vi "GraphsSandbox.vi"() -> ()   [LabVIEW 2016]
uses:
  <vilib>/Utility/miscctls.llb/LVOffsetAndMultiplierTypeDef.ctl
  <vilib>/measure/maresamp.llb/Resample Pair of Arrays (single shot).vi
  <userlib>/_OpenG.lib/array/array.llb/Empty 1D Array (DBL)__ogtk.vi
  <vilib>/measure/NI_MAPro.lvlib
  <vilib>/Analysis/NI_AALPro.lvlib
panel:
  in  "dt":dbl=1.0 format="%.2p"
  out "XY graphs 2":cluster{dbl[], dbl[]}[](graph)
  out "Numeric":i32
  out "antisymmetric":cluster{dbl[], dbl[]}[](graph)
  out "symmetric":cluster{dbl[], dbl[]}[](graph)
  out "line cuts":cluster{dbl[], dbl[]}[](graph)
  in  "y values to make line cuts":dbl[](array[numeric]) format="%#_6p"
  out "resampled intensity graph":dbl[][](graph)
  in  "XY graphs":cluster{dbl[], dbl[]}[](graph)
  in  "\"y\" array (each curve's parameter)":dbl[](array[numeric])=[1.0] format="%#_6p"
  # "1. convert x and y arrays to x and y scales for intensity graph"
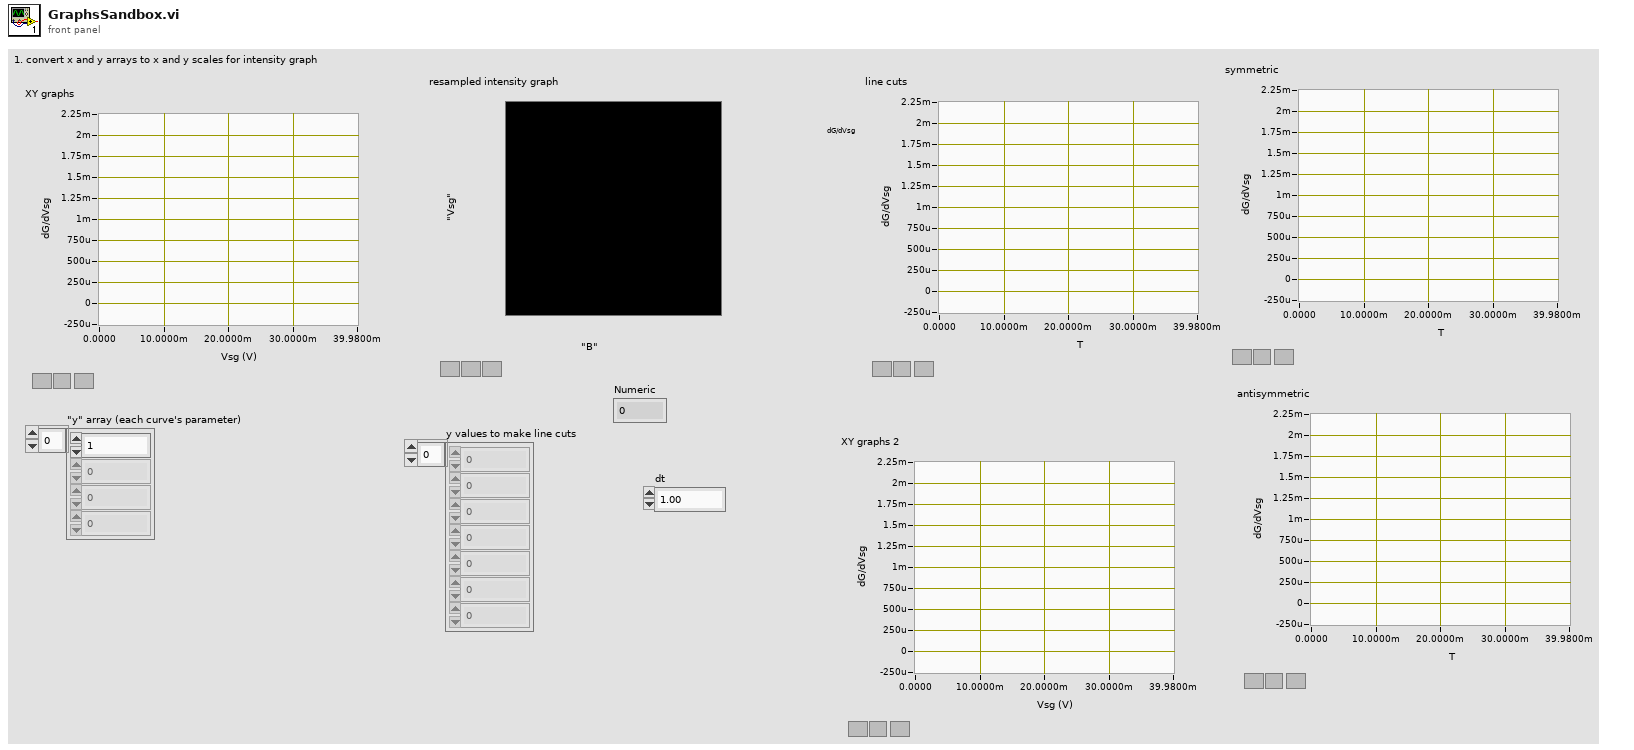
[diagram p1: front panel]
types:
  T1 = cluster{"x array":dbl[], "\"y\" array (parms)":dbl[], "XY graphs":cluster{dbl[], dbl[]}[]}
  T2 = typedef "LVOffsetAndMultiplierTypeDef.ctl" = cluster{"Offset":dbl, "Multiplier":dbl}
  T3 = cluster{"Decimated Array":dbl[], "Decimated Array":dbl[]}
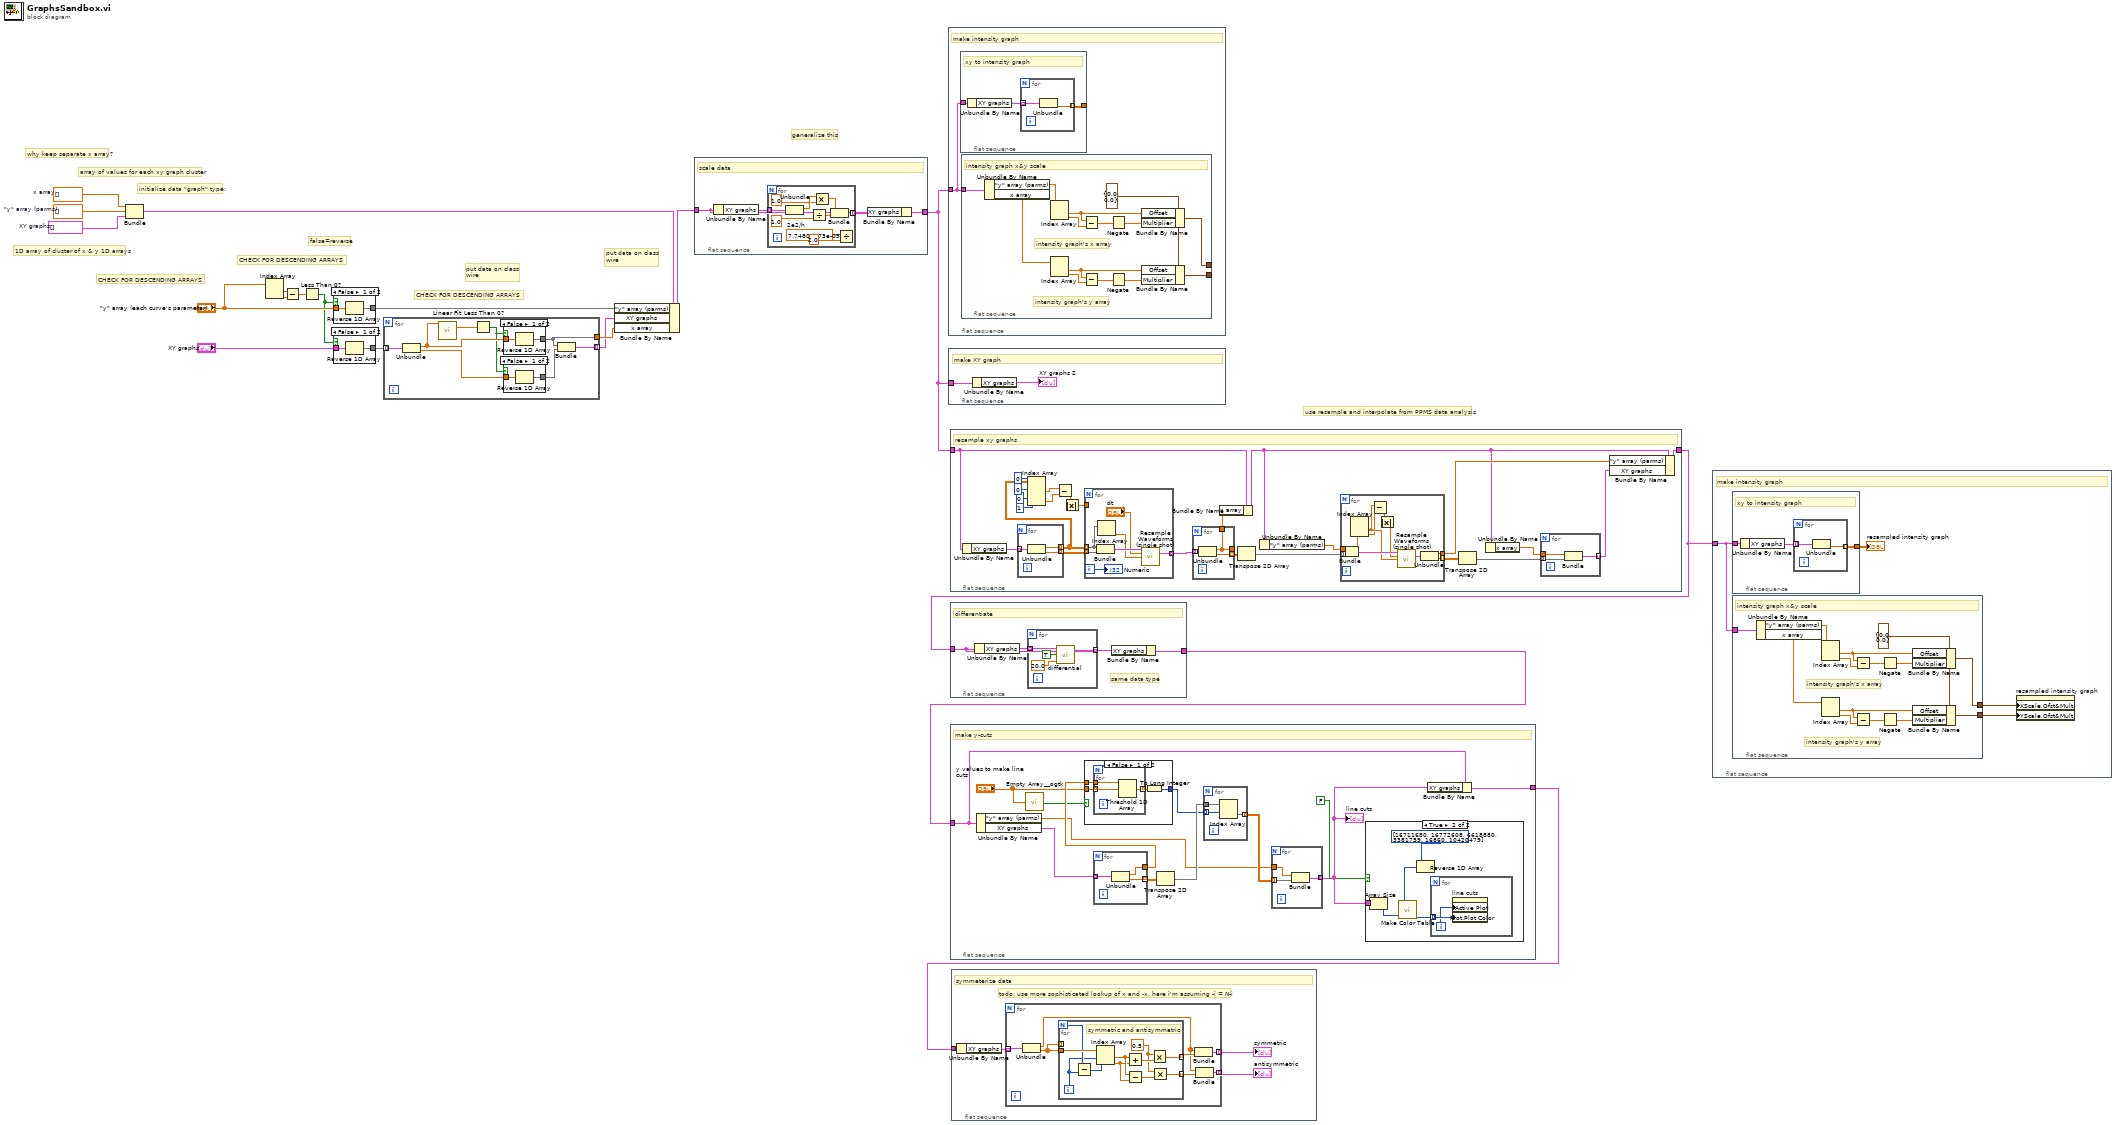
[diagram p0: block diagram]
diagram:
  w18 = dbl[] []  # x array
  w17 = cluster{dbl[], dbl[]}[] []  # XY graphs
  w19 = dbl[] []  # "y" array (parms)
  # "use resample and interpolate from PPMS data analysis"
  # "generalize this"
  # "array of values for each xy graph cluster"
  # "1D array of cluster of x & y 1D arrays"
  # "why keep separate x array?"
  # "CHECK FOR DESCENDING ARRAYS"
  # "false=reverse"
  # "put data on class\nwire"
  # "CHECK FOR DESCENDING ARRAYS"
  # "initialize data \"graph\" type:"
  # "CHECK FOR DESCENDING ARRAYS"
  # "put data on class\nwire"
  n1 = Bundle("x array"=w18, "\"y\" array (parms)"=w19, "XY graphs"=w17) -> (w16:T1)  [unwired: 1 in]
  n2 = Index Array(array="\"y\" array (each curve's parameter)") -> (element #1=w13:dbl, element #2=w14:dbl)  [unwired: 2 in]
  n3 = Subtract(x=w13, y=w14) -> (x-y=w12:dbl)
  n4 = Less Than 0?(x=w12) -> (x < 0?=w5:bool)
  n5 = case shown="False" w5 {
    tunnel: [w21 w22] -> w15
    tunnel: "\"y\" array (each curve's parameter)" -> [w20 w22]
    frame False {
      n6 = Reverse 1D Array(array=w20) -> (reversed array=w21:dbl[])
    }
    frame True {
    }
  }
  n7 = case shown="False" w5 {
    tunnel: [w24 w25] -> w6
    tunnel: "XY graphs" -> [w23 w25]
    frame False {
      n8 = Reverse 1D Array(array=w23) -> (reversed array=w24:cluster{dbl[], dbl[]}[])
    }
    frame True {
    }
  }
  n9 = for {
    tunnel: w6 -> [w33] mode=indexing
    tunnel: [w32] -> w10 mode=indexing
    tunnel: [w26] -> w11
    n10 = Unbundle(w33) -> (w30:dbl[], w28:dbl[])
    n11 = call <vilib>:"Linear Fit.vi"("Y"=w30) -> ("slope"=w31:dbl)  [unwired: 10 in, 4 out]
    n12 = Less Than 0?(x=w31) -> (x < 0?=w29:bool)
    n13 = case shown="False" w29 {
      tunnel: [w38 w39] -> w26
      tunnel: w30 -> [w37 w39]
      frame False {
        n14 = Reverse 1D Array(array=w37) -> (reversed array=w38:dbl[])
      }
      frame True {
      }
    }
    n15 = case shown="False" w29 {
      tunnel: [w35 w36] -> w27
      tunnel: w28 -> [w34 w36]
      frame False {
        n16 = Reverse 1D Array(array=w34) -> (reversed array=w35:dbl[])
      }
      frame True {
      }
    }
    n17 = Bundle(w26, w27) -> (w32:cluster{dbl[], dbl[]})  [unwired: 1 in]
  }
  n18 = Bundle By Name(cluster=w16, "\"y\" array (parms)"=w15, "XY graphs"=w10, "x array"=w11) -> (w9:T1)
  n19 = flat-sequence {
    tunnel: w9 -> [w41]
    tunnel: [w40] -> w4
    frame #0 {
      # "scale data"
      n20 = Unbundle By Name(w41) -> ("XY graphs"=w43:cluster{dbl[], dbl[]}[])
      n21 = for {
        tunnel: w43 -> [w53] mode=indexing
        tunnel: [w48] -> w42 mode=indexing
        w47 = 7.74809173e-05  # 2e2/h
        n22 = Unbundle(w53) -> (w50:dbl[], w52:dbl[])
        n23 = Divide(x=w52, y=1.0) -> (x/y=w51:dbl[])
        n24 = Multiply(x=w50, y=1.0) -> (x*y=w45:dbl[])
        n25 = Bundle(w45, w51) -> (w48:cluster{dbl[], dbl[]})  [unwired: 1 in]
        n26 = Divide(x=w47, y=2.0) -> ()  [unwired: 1 out]
      }
      n27 = Bundle By Name(cluster=w41, "XY graphs"=w42) -> (w40:T1)
    }
  }
  n28 = flat-sequence {
    tunnel: w4 -> [w54]
    frame #0 {
      # "make intensity graph"
      n29 = flat-sequence {
        tunnel: w54 -> [w70]
        tunnel: [w69] -> _
        frame #0 {
          # "xy to intensity graph"
          n30 = Unbundle By Name(w70) -> ("XY graphs"=w71:cluster{dbl[], dbl[]}[])
          n31 = for {
            tunnel: w71 -> [w73] mode=indexing
            tunnel: [w72] -> w69 mode=indexing
            n32 = Unbundle(w73) -> (w72:dbl[])  [unwired: 1 out]
          }
        }
      }
      n33 = flat-sequence {
        tunnel: [w68] -> _
        tunnel: [w58] -> _
        tunnel: w54 -> [w55]
        frame #0 {
          w59 = T2 {"Offset"=0.0, "Multiplier"=0.0} ("X Scale.Offset and Multiplier")
          # "intensity graph's y array"
          # "intensity graph's x array"
          # "intensity graph x&y scale"
          n34 = Unbundle By Name(w55) -> ("\"y\" array (parms)"=w57:dbl[], "x array"=w56:dbl[])
          n35 = Index Array(array=w57) -> (element #1=w62:dbl, element #2=w67:dbl)  [unwired: 2 in]
          n36 = Index Array(array=w56) -> (element #1=w60:dbl, element #2=w64:dbl)  [unwired: 2 in]
          n37 = Subtract(x=w62, y=w67) -> (x-y=w66:dbl)
          n38 = Subtract(x=w60, y=w64) -> (x-y=w65:dbl)
          n39 = Negate(x=w66) -> (-x=w63:dbl)
          n40 = Negate(x=w65) -> (-x=w61:dbl)
          n41 = Bundle By Name(cluster=w59, "Offset"=w62, "Multiplier"=w63) -> (w68:T2)
          n42 = Bundle By Name(cluster=w59, "Offset"=w60, "Multiplier"=w61) -> (w58:T2)
        }
      }
    }
  }
  n43 = flat-sequence {
    tunnel: w4 -> [w74]
    frame #0 {
      # "make XY graph"
      n44 = Unbundle By Name(w74) -> ("XY graphs"=→"XY graphs 2":cluster{dbl[], dbl[]}[])
    }
  }
  n45 = flat-sequence {
    tunnel: [w91] -> w2
    tunnel: w4 -> [w78]
    frame #0 {
      # "resample xy graphs"
      n46 = Unbundle By Name(w78) -> ("XY graphs"=w90:cluster{dbl[], dbl[]}[])
      n47 = for {
        tunnel: w90 -> [w102] mode=indexing
        tunnel: [w101] -> w89 mode=indexing
        tunnel: [w100] -> w84 mode=indexing
        n48 = Unbundle(w102) -> (w100:dbl[], w101:dbl[])
      }
      n49 = Index Array(array=w84, index (row) #1=0 ("index (row)"), index (col) #1=0 ("disabled index (col)"), index (row) #2=0 ("index (row)"), index (col) #2=1 ("disabled index (col)")) -> (element #1=w87:dbl, element #2=w85:dbl)
      n50 = Subtract(x=w87, y=w85) -> (x-y=w86:dbl)
      n51 = Absolute Value(x=w86) -> (abs(x)=w83:dbl)
      n52 = for {
        tunnel: w84 -> [w104] mode=indexing
        tunnel: w89 -> [w108] mode=indexing
        tunnel: [w107] -> w88 mode=indexing
        tunnel: w83 -> [_]
        i -> [w106]
        n53 = Bundle(w104, w108) -> (w109:cluster{dbl[], dbl[]})  [unwired: 1 in]
        n54 = Index Array(array=w104) -> (element=w103:dbl)  [unwired: 1 in]
        n55 = call-poly <vilib>:"Resample Waveforms (single shot).vi"("XY-data in"=w109, "dt"="dt", "t0"=w103) -> ("XY-data out"=w107:cluster{"X-array":dbl[], "Y-array":dbl[]})  [unwired: 8 in, 4 out]
        "Numeric" <- w106
      }
      n56 = for {
        tunnel: w88 -> [w112] mode=indexing
        tunnel: [w111] -> w96 mode=indexing
        tunnel: [w110] -> _
        tunnel: [w110] -> w77
        n57 = Unbundle(w112) -> ("X-array"=w110:dbl[], "Y-array"=w111:dbl[])
      }
      n58 = Bundle By Name(cluster=w78, "x array"=w77) -> (w76:T1)
      n59 = Transpose 2D Array(2D array=w96) -> (transposed array=w99:dbl[][])
      n60 = Unbundle By Name(w76) -> ("\"y\" array (parms)"=w95:dbl[])
      n61 = for {
        tunnel: w99 -> [w125] mode=indexing
        tunnel: w95 -> [w123]
        tunnel: [w120] -> w98 mode=indexing
        tunnel: [w119] -> w93
        n62 = Bundle("\"y\" array (parms)"=w123, w125) -> (w124:cluster{"\"y\" array (parms)":dbl[], dbl[]})  [unwired: 1 in]
        n63 = Index Array(array=w123) -> (element #1=w122:dbl, element #2=w121:dbl)  [unwired: 2 in]
        n64 = Subtract(x=w122, y=w121) -> (x-y=w117:dbl)
        n65 = Absolute Value(x=w117) -> (abs(x)=w116:dbl)
        n66 = call-poly <vilib>:"Resample Waveforms (single shot).vi"("XY-data in"=w124, "dt"=w116, "t0"=w122) -> ("XY-data out"=w118:cluster{"X-array":dbl[], "Y-array":dbl[]})  [unwired: 8 in, 4 out]
        n67 = Unbundle(w118) -> ("X-array"=w119:dbl[], "Y-array"=w120:dbl[])
      }
      n68 = Transpose 2D Array(2D array=w98) -> (transposed array=w97:dbl[][])
      n69 = Unbundle By Name(w76) -> ("x array"=w94:dbl[])
      n70 = for {
        tunnel: w97 -> [w115] mode=indexing
        tunnel: w94 -> [w114]
        tunnel: [w113] -> w92 mode=indexing
        n71 = Bundle("x array"=w114, w115) -> (w113:cluster{"x array":dbl[], dbl[]})  [unwired: 1 in]
      }
      n72 = Bundle By Name(cluster=w76, "\"y\" array (parms)"=w93, "XY graphs"=w92) -> (w91:T1)
    }
  }
  n73 = flat-sequence {
    tunnel: [w127] -> w3
    tunnel: w2 -> [w126]
    frame #0 {
      # "same data type"
      # "differentiate"
      n74 = Unbundle By Name(w126) -> ("XY graphs"=w128:cluster{dbl[], dbl[]}[])
      n75 = for {
        tunnel: w128 -> [w133] mode=indexing
        tunnel: [w130] -> w129 mode=indexing
        n76 = call <userlib>:"differential.vi"("Numeric"=20.0, "dy/dx vs x"=TRUE, "A vs B 2"=w133) -> ("A vs B 3"=w130:T3)  [unwired: 1 in]
      }
      n77 = Bundle By Name(cluster=w126, "XY graphs"=w129) -> (w127:T1)
    }
  }
  n78 = flat-sequence {
    tunnel: w3 -> [w136]
    tunnel: [w134] -> w1
    frame #0 {
      # "make y-cuts"
      n79 = Unbundle By Name(w136) -> ("\"y\" array (parms)"=w140:dbl[], "XY graphs"=w146:cluster{dbl[], dbl[]}[])
      n80 = call-poly <userlib>:"Empty Array__ogtk.vi"("Array"="y values to make line cuts") -> ("Empty Array?"=w138:bool)  [unwired: 8 in]
      n81 = for {
        tunnel: w146 -> [w172] mode=indexing
        tunnel: [w171] -> w145 mode=indexing
        tunnel: [w170] -> w141
        n82 = Unbundle(w172) -> (w170:dbl[], w171:dbl[])
      }
      n83 = case shown="False" w138 {
        tunnel: [w154 w161] -> w143
        tunnel: w141 -> [w156 w162]
        tunnel: "y values to make line cuts" -> [w155 _]
        frame False {
          n84 = for {
            tunnel: w156 -> [w160]
            tunnel: w155 -> [w159] mode=indexing
            tunnel: [w158] -> w157 mode=indexing
            n85 = Threshold 1D Array(2:w159, 3:w160) -> (0:w158:dbl)  [unwired: 1 in]
          }
          n86 = To Long Integer(number=w157) -> (32bit integer=w154:i32[])
        }
        frame True {
          n87 = for {
            tunnel: w162 -> [_] mode=indexing
            tunnel: [w163] -> w161 mode=indexing
            i -> [w163]
          }
        }
      }
      n88 = Transpose 2D Array(2D array=w145) -> (transposed array=w144:dbl[][])
      n89 = for {
        tunnel: w144 -> [w169]
        tunnel: w143 -> [w168] mode=indexing
        tunnel: [w167] -> w142 mode=indexing
        n90 = Index Array(array=w169, index (row)=w168) -> (element=w167:dbl[])  [unwired: 1 in]
      }
      n91 = for {
        tunnel: w142 -> [w166] mode=indexing
        tunnel: w140 -> [w165]
        tunnel: [w164] -> w135 mode=indexing
        n92 = Bundle("\"y\" array (parms)"=w165, w166) -> (w164:cluster{"\"y\" array (parms)":dbl[], dbl[]})  [unwired: 1 in]
      }
      "line cuts" <- w135
      n93 = case shown="True" FALSE {
        tunnel: w135 -> [_ w147]
        frame False {
        }
        frame True {
          n94 = Array Size(array=w147) -> (size(s)=w151:i32)
          n95 = Reverse 1D Array(array=u32[] [16711680, 16772608, 6618880, 3381759, 16860, 10420479] ("color scale")) -> (reversed array=w148:u32[])
          n96 = call <userlib>:"Make Color Table.vi"("Array"=w148, "Size/3"=w151) -> ("Color Tbl"=w149:u32[])  [unwired: 3 out]
          n97 = for {
            tunnel: w149 -> [w153] mode=indexing
            i -> [w152]
            n98 = property on="line cuts" class="XYGraph (strict)"("Active Plot"=w152, "Plot.Plot Color"=w153) -> ()  [unwired: 2 in, 2 out]
          }
        }
      }
      n99 = Bundle By Name(cluster=w136, "XY graphs"=w135) -> (w134:T1)
    }
  }
  n100 = flat-sequence {
    tunnel: w1 -> [w174]
    frame #0 {
      # "todo: use more sophisticated lookup of x and -x. here i'm assuming -i = N-i"
      # "symmeterize data"
      n101 = Unbundle By Name(w174) -> ("XY graphs"=w173:cluster{dbl[], dbl[]}[])
      n102 = for {
        tunnel: w173 -> [w183] mode=indexing
        tunnel: [w178] -> w176 mode=indexing
        tunnel: [w177] -> w175 mode=indexing
        n103 = Unbundle(w183) -> (w179:dbl[], w182:dbl[])
        n104 = for {
          N -> [w193]
          tunnel: w182 -> [w194]
          tunnel: w182 -> [_] mode=indexing
          tunnel: [w185] -> w181 mode=indexing
          tunnel: [w184] -> w180 mode=indexing
          i -> [w192]
          w186 = 0.5 ("x")
          # "symmetric and antisymmetric"
          n105 = Subtract(x=w193, y=w192) -> (x-y=w191:i32)
          n106 = Index Array(array=w194, index #1=w192, index #2=w191) -> (element #1=w190:dbl, element #2=w189:dbl)
          n107 = Add(x=w190, y=w189) -> (x+y=w188:dbl)
          n108 = Subtract(x=w190, y=w189) -> (x-y=w187:dbl)
          n109 = Multiply(x=w186, y=w188) -> (x*y=w185:dbl)
          n110 = Multiply(x=w186, y=w187) -> (x*y=w184:dbl)
        }
        n111 = Bundle(w179, w181) -> (w178:cluster{dbl[], dbl[]})  [unwired: 1 in]
        n112 = Bundle(w179, w180) -> (w177:cluster{dbl[], dbl[]})  [unwired: 1 in]
      }
      "antisymmetric" <- w175
      "symmetric" <- w176
    }
  }
  n113 = flat-sequence {
    tunnel: w2 -> [w195]
    frame #0 {
      # "make intensity graph"
      n114 = flat-sequence {
        tunnel: [w214] -> w198
        tunnel: w195 -> [w213]
        frame #0 {
          # "xy to intensity graph"
          n115 = Unbundle By Name(w213) -> ("XY graphs"=w215:cluster{dbl[], dbl[]}[])
          n116 = for {
            tunnel: w215 -> [w217] mode=indexing
            tunnel: [w216] -> w214 mode=indexing
            n117 = Unbundle(w217) -> (w216:dbl[])  [unwired: 1 out]
          }
        }
      }
      n118 = flat-sequence {
        tunnel: [w212] -> w197
        tunnel: [w202] -> w196
        tunnel: w195 -> [w199]
        frame #0 {
          w203 = T2 {"Offset"=0.0, "Multiplier"=0.0} ("X Scale.Offset and Multiplier")
          # "intensity graph's y array"
          # "intensity graph's x array"
          # "intensity graph x&y scale"
          n119 = Unbundle By Name(w199) -> ("\"y\" array (parms)"=w201:dbl[], "x array"=w200:dbl[])
          n120 = Index Array(array=w201) -> (element #1=w206:dbl, element #2=w211:dbl)  [unwired: 2 in]
          n121 = Index Array(array=w200) -> (element #1=w204:dbl, element #2=w208:dbl)  [unwired: 2 in]
          n122 = Subtract(x=w206, y=w211) -> (x-y=w210:dbl)
          n123 = Subtract(x=w204, y=w208) -> (x-y=w209:dbl)
          n124 = Negate(x=w210) -> (-x=w207:dbl)
          n125 = Negate(x=w209) -> (-x=w205:dbl)
          n126 = Bundle By Name(cluster=w203, "Offset"=w206, "Multiplier"=w207) -> (w212:T2)
          n127 = Bundle By Name(cluster=w203, "Offset"=w204, "Multiplier"=w205) -> (w202:T2)
        }
      }
      n128 = property on="resampled intensity graph" class="IntGraph (strict)"("XScale.Ofst&Mult"=w197, "YScale.Ofst&Mult"=w196) -> ()  [unwired: 2 in, 2 out]
      "resampled intensity graph" <- w198
    }
  }
